vi "AudioTest.Calibrate Generated Waveform, Read Waveform Config File.vi"(8 "error in":errorcluster, 10 "Power Scale":bool=TRUE, 11 "Config File":path=path "C:/Github/Valve/MTE-Testers-LV2018/MTE Testers/HMD/Audio Test/Config/Speaker Calibration, PN XXX, SN YYY, v10-30-18.csv") -> (0 "error out":errorcluster, 3 "Waveform Cal":cluster{"Freq":dbl[], "Gain":dbl[]})   [LabVIEW 2018]
uses:
  <vilib>/KATE/Files/File Utils.lvlib
panel:
  out "1/Avg G Norm":dbl
  out "1/Min G Norm":dbl
  out "Min G Norm":dbl
  out "Max G Norm":dbl
  out "1/Min G":dbl
  out "Min G":dbl
  out "Max G":dbl
  out "Cal Data Amplitude":cluster{"Freq":dbl[], "Gain":dbl[]}(graph)
  out "1/Amplitude Multiplier":cluster{"Freq":dbl[], "Gain":dbl[]}(graph)
  out "Amplitude Multiplier":cluster{"Freq":dbl[], "Gain":dbl[]}(graph)
  out "Cal Data":cluster{"Freq":dbl[], "Gain":dbl[]}(graph)
  out "Normalized":cluster{"Freq":dbl[], "Gain":dbl[]}(graph)
  out "XY Graph":cluster{"Freq":dbl[], "Gain":dbl[]}(graph)
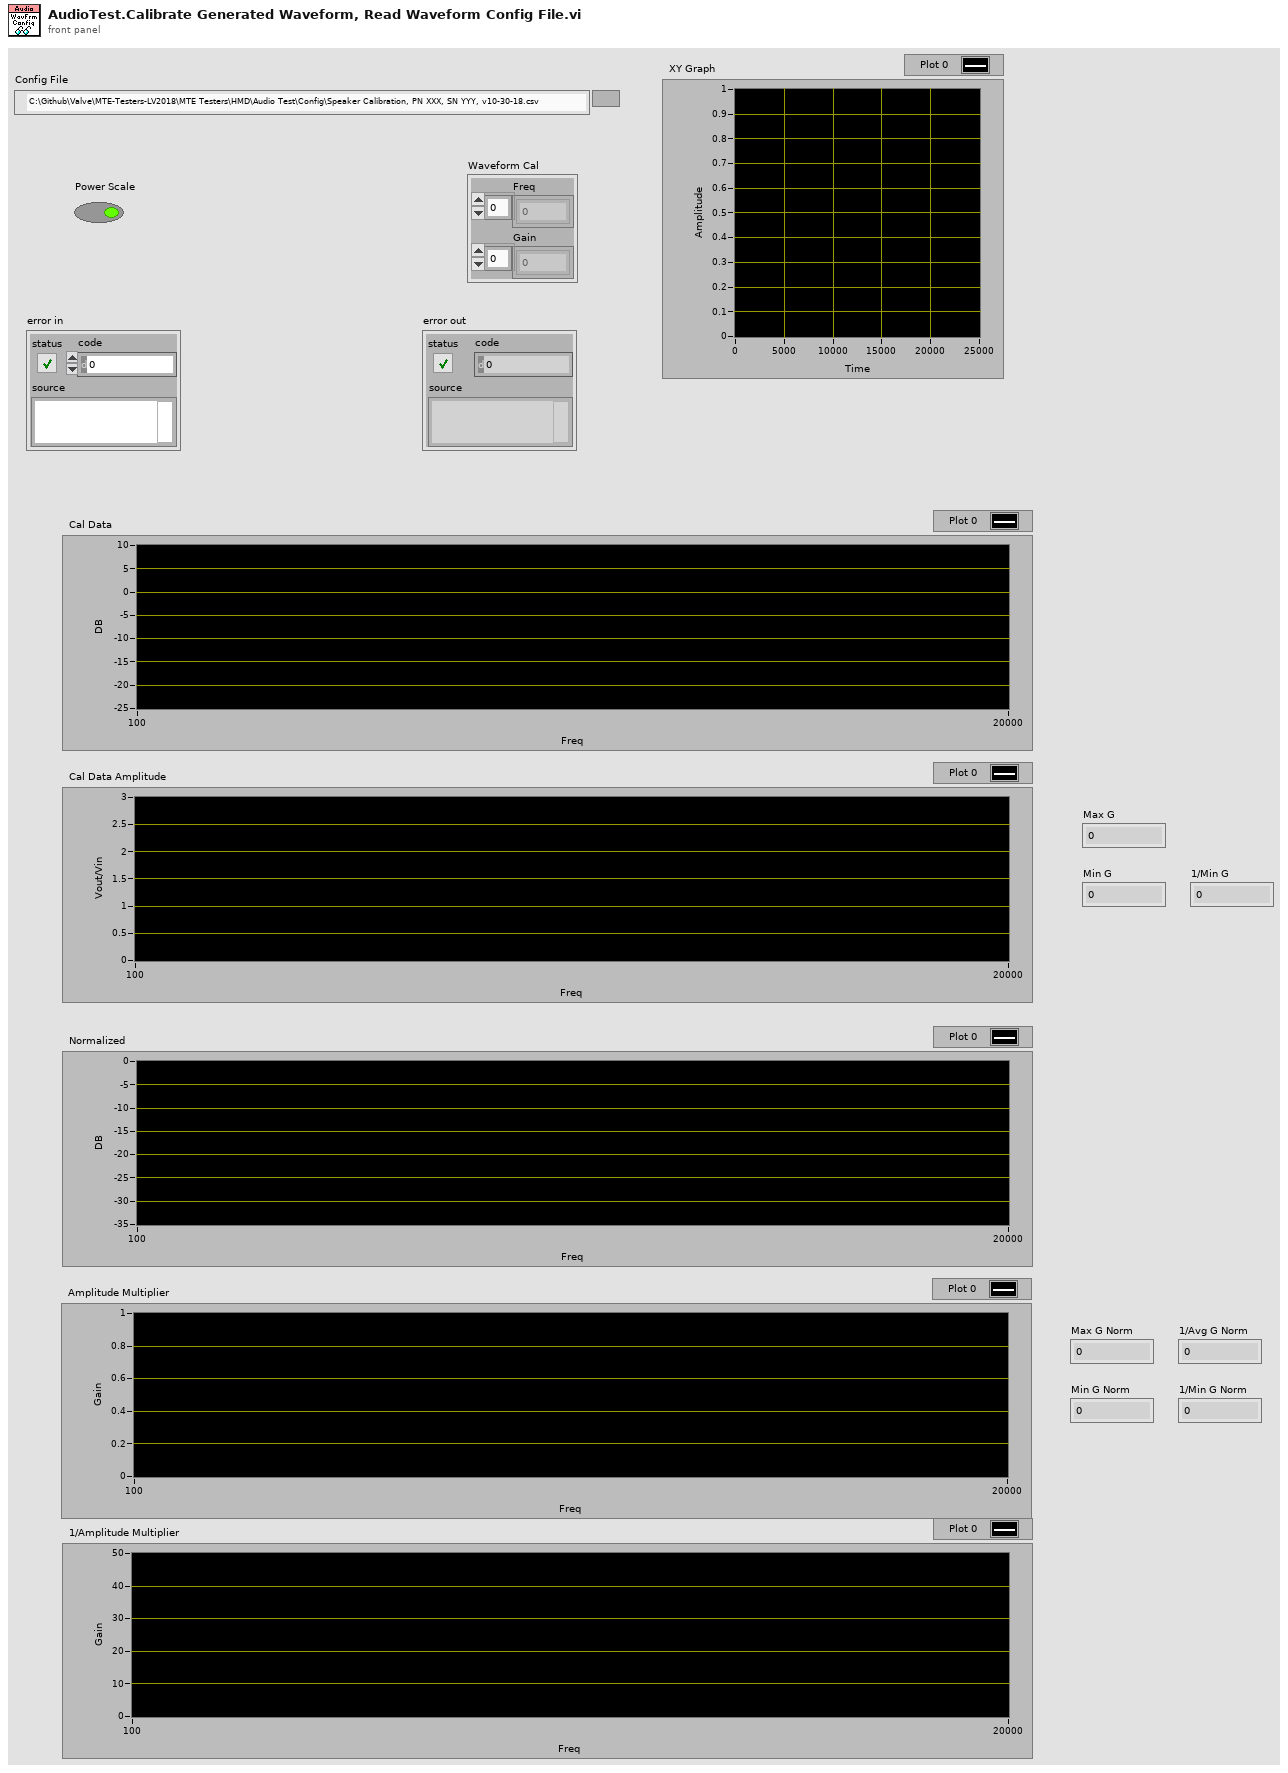
[diagram p1: front panel]
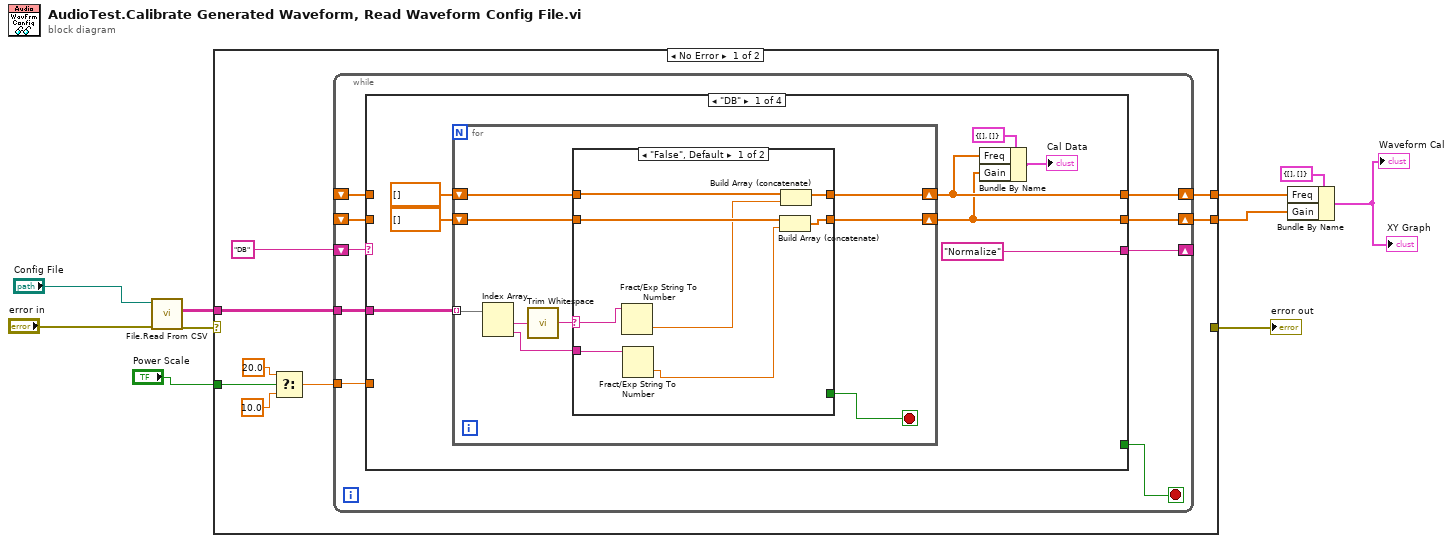
[diagram p0: block diagram]
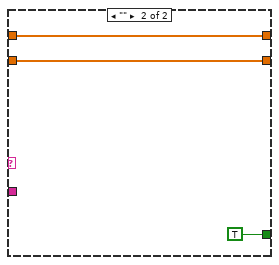
[diagram p2: hidden frame]
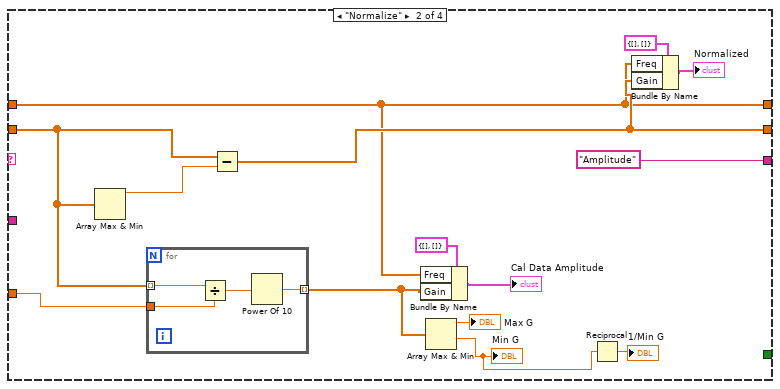
[diagram p3: hidden frame]
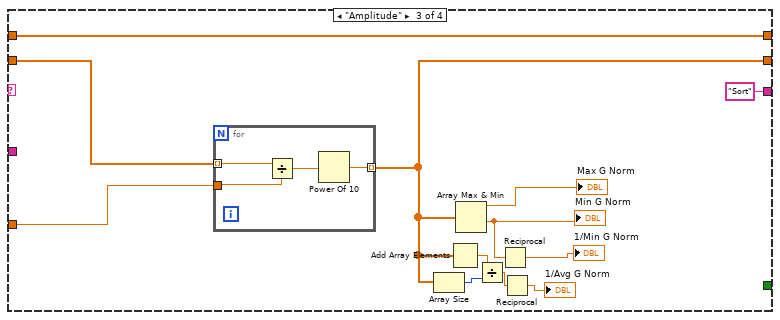
[diagram p4: hidden frame]
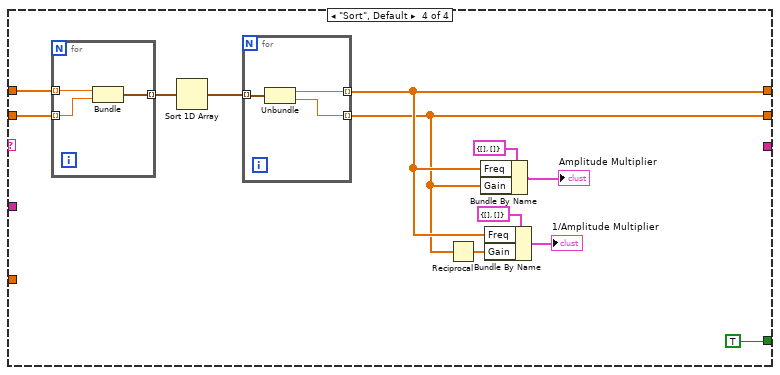
[diagram p5: hidden frame]
diagram:
  n1 = call <vilib>:"File.Read From CSV.vi"("error in"="error in", "File"="Config File") -> ("error out"=w7:errorcluster, "Data"=w8:string[][])  [unwired: 7 in, 1 out]
  n2 = case shown="No Error" w7 {
    selector: w7 -> [_ w108]
    tunnel: w8 -> [w18 _]
    tunnel: [_ w108] -> w6
    tunnel: [w17 _] -> w4
    tunnel: [w16 _] -> w3
    tunnel: "Power Scale" -> [w12 _]
    frame No Error {
      n3 = Select(t=20.0 ("y"), s=w12, f=10.0 ("y")) -> (s? t:f=w11:dbl)
      n4 = while {
        tunnel: w18 -> [w27]
        shift-right: [w21] -> _
        shift-left: "DB" -> [w24]
        shift-right: [w25] -> w16
        shift-left: _ -> [w22]
        shift-right: [w26] -> w17
        shift-left: _ -> [w23]
        tunnel: w11 -> [w19]
        stop <- w20 stop-if-true
        n5 = case shown="\"DB\"" w24 {
          tunnel: w27 -> [w35 _ _ _]
          tunnel: [w30 w62 w84 w91] -> w26
          tunnel: [w29 w65 w77 w90] -> w25
          tunnel: w23 -> [_ w62 w84 w100]
          tunnel: w22 -> [_ w64 w85 w99]
          tunnel: ["Normalize" "Amplitude" "Sort" _] -> w21
          tunnel: [_ _ _ TRUE] -> w20
          tunnel: w19 -> [_ w60 w83 _]
          frame "DB" {
            n6 = for {
              tunnel: w35 -> [w44] mode=indexing
              shift-right: [w38] -> w30
              shift-left: dbl[] [] ("X") -> [w40]
              shift-right: [w37] -> w29
              shift-left: dbl[] [] ("Y") -> [w39]
              stop <- w41 stop-if-true
              n7 = Index Array(array=w44) -> (element #1=w43:string, element #2=w36:string)  [unwired: 2 in]
              n8 = call <vilib>:"Trim Whitespace.vi"("string"=w43) -> ("trimmed string"=w42:string)  [unwired: 1 in]
              n9 = case shown="\"False\", Default" w42 {
                selector: w42 -> [w51 _]
                tunnel: [_ TRUE] -> w41
                tunnel: w40 -> [w47 w54]
                tunnel: w39 -> [w50 w53]
                tunnel: [w48 w54] -> w38
                tunnel: [w49 w53] -> w37
                tunnel: w36 -> [w52 _]
                frame "False", Default {
                  n10 = Fract/Exp String To Number(string=w51) -> (number=w46:dbl)  [unwired: 3 in, 1 out]
                  n11 = Fract/Exp String To Number(string=w52) -> (number=w45:dbl)  [unwired: 3 in, 1 out]
                  n12 = Build Array (concatenate)(w50, w45) -> (w49:dbl[])
                  n13 = Build Array (concatenate)(w47, w46) -> (w48:dbl[])
                }
                frame "" {
                }
              }
            }
            n14 = Bundle By Name(cluster=cluster{"Freq":dbl[], "Gain":dbl[]} {"Freq"=[], "Gain"=[]} ("Waveform Cal"), "Freq"=w30, "Gain"=w29) -> (→"Cal Data":cluster{"Freq":dbl[], "Gain":dbl[]})
          }
          frame "Normalize" {
            n15 = Array Max & Min(array=w64) -> (max value=w68:dbl)  [unwired: 3 out]
            n16 = for {
              tunnel: w64 -> [w72] mode=indexing
              tunnel: [w71] -> w59 mode=indexing
              tunnel: w60 -> [w70]
              n17 = Divide(x=w72, y=w70) -> (x/y=w73:dbl)
              n18 = Power Of 10(x=w73) -> (10^x=w71:dbl)
            }
            n19 = Subtract(x=w64, y=w68) -> (x-y=w65:dbl[])
            n20 = Bundle By Name(cluster=cluster{"Freq":dbl[], "Gain":dbl[]} {"Freq"=[], "Gain"=[]} ("Waveform Cal"), "Freq"=w62, "Gain"=w59) -> (→"Cal Data Amplitude":cluster{"Freq":dbl[], "Gain":dbl[]})
            n21 = Array Max & Min(array=w59) -> (max value=→"Max G":dbl, min value=w56:dbl)  [unwired: 2 out]
            "Min G" <- w56
            n22 = Reciprocal(x=w56) -> (1/x=→"1/Min G":dbl)
            n23 = Bundle By Name(cluster=cluster{"Freq":dbl[], "Gain":dbl[]} {"Freq"=[], "Gain"=[]} ("Waveform Cal"), "Freq"=w62, "Gain"=w65) -> (→"Normalized":cluster{"Freq":dbl[], "Gain":dbl[]})
          }
          frame "Amplitude" {
            n24 = for {
              tunnel: w85 -> [w88] mode=indexing
              tunnel: [w87] -> w77 mode=indexing
              tunnel: w83 -> [w86]
              n25 = Divide(x=w88, y=w86) -> (x/y=w89:dbl)
              n26 = Power Of 10(x=w89) -> (10^x=w87:dbl)
            }
            n27 = Array Size(array=w77) -> (size(s)=w78:i32)
            n28 = Add Array Elements(numeric array=w77) -> (sum=w79:dbl)
            n29 = Array Max & Min(array=w77) -> (max value=→"Max G Norm":dbl, min value=w81:dbl)  [unwired: 2 out]
            "Min G Norm" <- w81
            n30 = Divide(x=w79, y=w78) -> (x/y=w76:dbl)
            n31 = Reciprocal(x=w81) -> (1/x=→"1/Min G Norm":dbl)
            n32 = Reciprocal(x=w76) -> (1/x=→"1/Avg G Norm":dbl)
          }
          frame "Sort", Default {
            n33 = for {
              tunnel: w100 -> [w107] mode=indexing
              tunnel: w99 -> [w106] mode=indexing
              tunnel: [w105] -> w98 mode=indexing
              n34 = Bundle(w107, w106) -> (w105:cluster{dbl, dbl})  [unwired: 1 in]
            }
            n35 = Sort 1D Array(array=w98) -> (sorted array=w97:cluster{dbl, dbl}[])
            n36 = for {
              tunnel: w97 -> [w104] mode=indexing
              tunnel: [w103] -> w91 mode=indexing
              tunnel: [w102] -> w90 mode=indexing
              n37 = Unbundle(w104) -> (w103:dbl, w102:dbl)
            }
            n38 = Reciprocal(x=w90) -> (1/x=w93:dbl[])
            n39 = Bundle By Name(cluster=cluster{"Freq":dbl[], "Gain":dbl[]} {"Freq"=[], "Gain"=[]} ("Waveform Cal"), "Freq"=w91, "Gain"=w90) -> (→"Amplitude Multiplier":cluster{"Freq":dbl[], "Gain":dbl[]})
            n40 = Bundle By Name(cluster=cluster{"Freq":dbl[], "Gain":dbl[]} {"Freq"=[], "Gain"=[]} ("Waveform Cal"), "Freq"=w91, "Gain"=w93) -> (→"1/Amplitude Multiplier":cluster{"Freq":dbl[], "Gain":dbl[]})
          }
        }
      }
    }
    frame Error {
    }
  }
  "error out" <- w6
  n41 = Bundle By Name(cluster=cluster{"Freq":dbl[], "Gain":dbl[]} {"Freq"=[], "Gain"=[]} ("Waveform Cal"), "Freq"=w4, "Gain"=w3) -> (→"Waveform Cal" →"XY Graph":cluster{"Freq":dbl[], "Gain":dbl[]})
